vi "multiple_ScopeTRace_FGV.vi"(9 "output cluster 2":T1, 10 "Nr.":i32, 11 "command":T2=enum."get ALL") -> (1 "output cluster 2":T1)   [LabVIEW 2013]
uses:
  commandForScopeTrace.ctl
  scopeTrace_TypDef.ctl
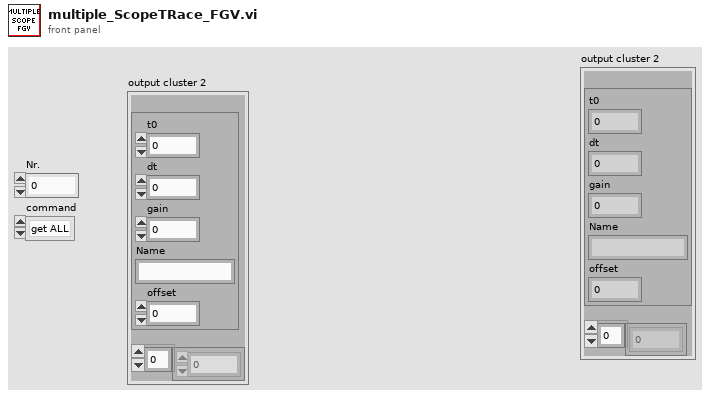
[diagram p1: front panel]
types:
  T1 = typedef "scopeTrace_TypDef.ctl" = cluster{"Info":cluster{"t0":dbl, "dt":dbl, "gain":dbl, "Name":string, "offset":dbl}, "Data":i16[]}
  T2 = typedef "commandForScopeTrace.ctl" = enum16{"get", "set", "init", "get ALL"}
  T3 = typedef "scopeTrace_TupDef.ctl" = cluster{cluster{"t0":dbl, "dt":dbl, "gain":dbl, "Name":string, "offset":dbl}, i16[]}
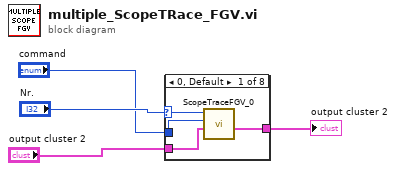
[diagram p0: block diagram]
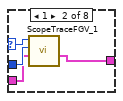
[diagram p2: hidden frame]
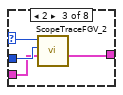
[diagram p3: hidden frame]
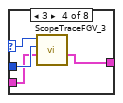
[diagram p4: hidden frame]
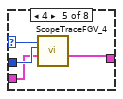
[diagram p5: hidden frame]
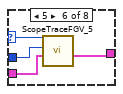
[diagram p6: hidden frame]
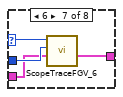
[diagram p7: hidden frame]
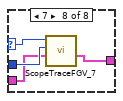
[diagram p8: hidden frame]
diagram:
  n1 = case shown="0, Default" "Nr." {
    selector: "Nr." -> [w8 w12 w16 w20 w24 w28 w32 w36]
    tunnel: "command" -> [w7 w11 w15 w19 w23 w27 w31 w35]
    tunnel: "output cluster 2" -> [w6 w10 w14 w18 w22 w26 w30 w34]
    tunnel: [w5 w9 w13 w17 w21 w25 w29 w33] -> w1
    frame 0, Default {
      n2 = call "ScopeTraceFGV_0.vi"("output cluster 2"=w6, "command"=w7, "Nr."=w8) -> ("output cluster 2"=w5:T3)  [unwired: 8 in]
    }
    frame 1 {
      n3 = call "ScopeTraceFGV_1.vi"("output cluster 2"=w10, "command"=w11, "Nr."=w12) -> ("output cluster 2"=w9:T3)  [unwired: 8 in]
    }
    frame 2 {
      n4 = call "ScopeTraceFGV_2.vi"("output cluster 2"=w14, "command"=w15, "Nr."=w16) -> ("output cluster 2"=w13:T3)  [unwired: 8 in]
    }
    frame 3 {
      n5 = call "ScopeTraceFGV_3.vi"("output cluster 2"=w18, "command"=w19, "Nr."=w20) -> ("output cluster 2"=w17:T3)  [unwired: 8 in]
    }
    frame 4 {
      n6 = call "ScopeTraceFGV_4.vi"("output cluster 2"=w22, "command"=w23, "Nr."=w24) -> ("output cluster 2"=w21:T3)  [unwired: 8 in]
    }
    frame 5 {
      n7 = call "ScopeTraceFGV_5.vi"("output cluster 2"=w26, "command"=w27, "Nr."=w28) -> ("output cluster 2"=w25:T3)  [unwired: 8 in]
    }
    frame 6 {
      n8 = call "ScopeTraceFGV_6.vi"("output cluster 2"=w30, "command"=w31, "Nr."=w32) -> ("output cluster 2"=w29:T3)  [unwired: 8 in]
    }
    frame 7 {
      n9 = call "ScopeTraceFGV_7.vi"("output cluster 2"=w34, "command"=w35, "Nr."=w36) -> ("output cluster 2"=w33:T3)  [unwired: 8 in]
    }
  }
  "output cluster 2" <- w1
